vi "VGI Reset Pins.vi"(9 "PinMask":u16, 10 "DevIndex":i32, 11 "DevType":i32) -> (3 "function return":i32)   [LabVIEW 2010, in "ControlGPIO.lvlib"]
doc: "int WINAPI VGI_ResetPins(int DevType,int DevIndex,unsigned short PinMask);"
uses:
  ControlGPIO.lvlib
  ControlGPIO/Ginkgo_Driver.dll
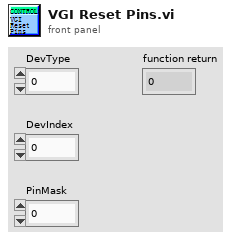
[diagram p1: front panel]
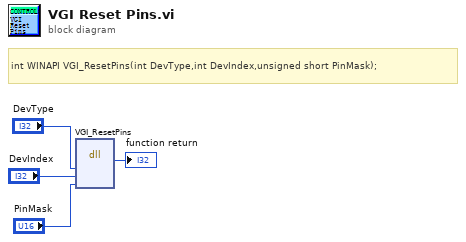
[diagram p0: block diagram]
diagram:
  # "int\tWINAPI VGI_ResetPins(int DevType,int DevIndex,unsigned short PinMask);"
  n1 = dll-call lib="E:/Project/vt_ginkgo/truck/Ginkgo Driver/vs2010/Ginkgo_USB-I2C&SPI&CAN_API_v2.0.3.3/lib/labview_32bit/ControlGPIO/Ginkgo_Driver.*" fn="VGI_ResetPins"("DevType"="DevType", "DevIndex"="DevIndex", "PinMask"="PinMask") -> (→"function return":i32)  [unwired: 6 in, 2 out]
